vi "Vision_Overlays.vi"(6 "Center":T2, 7 "Bounding Box":cluster{"X":dbl, "Y":dbl}[](array[cluster]), 8 "error in (no error)":errorcluster, 9 "Destination":T2, 10 "Position":cluster{"X":dbl, "Y":dbl}, 11 "Image in":T1) -> (0 "error out":errorcluster, 3 "Image out":T1)   [LabVIEW 2017]
doc: "Overlay points, lines and text on the image."
uses:
  <vilib>/vision/Image Controls.llb/IMAQ Image.ctl
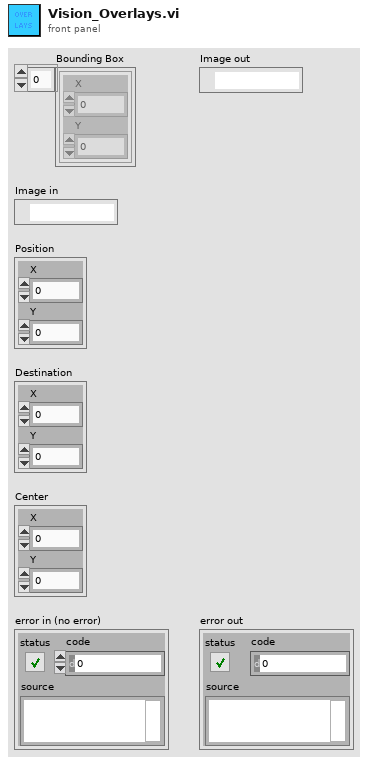
[diagram p1: front panel]
types:
  T1 = typedef "IMAQ Image.ctl" = refnum<image>
  T2 = typedef "IMAQ Point" = cluster{"X":sgl, "Y":sgl}
  T3 = cluster{"Desired Font (Application)":enum16{"User-specified Font", "Application Font", "System Font", "Dialog Font"}, "[User-specified Font]":cluster{"Font Name":string, "Size":i16, "Strikeout?":bool, "Italic?":bool, "Underline?":bool, "Outline?":bool, "Shadow?":bool, "Bold?":bool, "Rotation Angle":dbl}, "Horizontal Alignment":i16, "Vertical Alignment":i16}
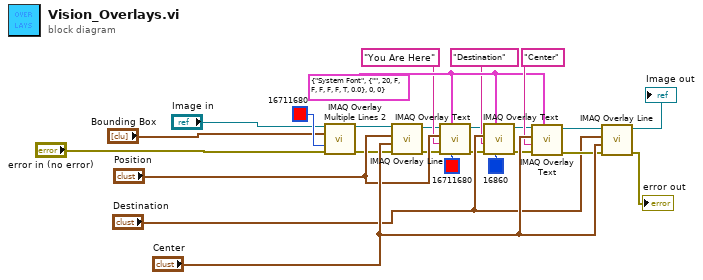
[diagram p0: block diagram]
diagram:
  w21 = T3 {"Desired Font (Application)"=enum."System Font", "[User-specified Font]"={"Font Name"="", "Size"=20, "Strikeout?"=FALSE, "Italic?"=FALSE, "Underline?"=FALSE, "Outline?"=FALSE, "Shadow?"=FALSE, "Bold?"=TRUE, "Rotation Angle"=0.0}, "Horizontal Alignment"=0, "Vertical Alignment"=0} ("Font, Size & Style")
  n1 = call "IMAQ Overlay Multiple Lines 2"("Image"="Image in", "Line End Points"="Bounding Box", "Color"=u32 16711680, "error in (no error)"="error in (no error)") -> ("Image Out"=w25:T1, "error out"=w5:errorcluster)  [unwired: 4 in, 6 out]
  n2 = call "IMAQ Overlay Line"("error in (no error)"=w5, "End Point"="Center", "Start Point"="Position", "Image"=w25) -> ("error out"=w11:errorcluster, "Image Out"=w10:T1)  [unwired: 6 in]
  n3 = call "IMAQ Overlay Text"("Text Color (black)"=u32 16711680, "Font, Size & Style"=w21, "error in (no error)"=w11, "String"="You Are Here", "Origin"="Position", "Image"=w10) -> ("error out"=w8:errorcluster, "Image Out"=w9:T1)  [unwired: 4 in]
  n4 = call "IMAQ Overlay Text"("Text Color (black)"=u32 16860, "Font, Size & Style"=w21, "error in (no error)"=w8, "String"="Destination", "Origin"="Destination", "Image"=w9) -> ("error out"=w17:errorcluster, "Image Out"=w18:T1)  [unwired: 4 in]
  n5 = call "IMAQ Overlay Text"("Font, Size & Style"=w21, "error in (no error)"=w17, "String"="Center", "Origin"="Center", "Image"=w18) -> ("error out"=w19:errorcluster, "Image Out"=w20:T1)  [unwired: 5 in]
  n6 = call "IMAQ Overlay Line"("error in (no error)"=w19, "End Point"="Center", "Start Point"="Destination", "Image"=w20) -> ("error out"=→"error out":errorcluster, "Image Out"=→"Image out":T1)  [unwired: 6 in]
